vi "GLdrv_FILE_TRANS_SOUR.vi"(0 "Connection ID":T1, 5 "File Path":string, 11 "error in (no error)":errorcluster, 13 "Query(f)":bool) -> (4 "Connection ID Out":T1, 6 "File Path out":string, 15 "error out":errorcluster)   [LabVIEW 2017, in "GL860_Driver.lvlib"]
doc: "記録計本体内のファイルを転送します\nファイルの設定を行います\n例）　:FILE:TRNAS:SOUR \"MEM\\FOLDER\\ABCD.GBD”"
uses:
  GL860_Driver.lvlib
  ConnectionID.ctl
  GLdrv_RW.ctl
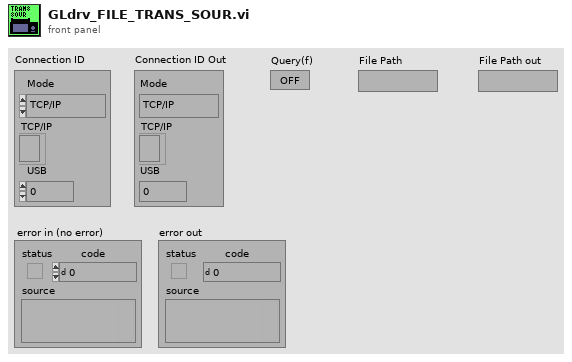
[diagram p1: front panel]
types:
  T1 = typedef "ConnectionID.ctl" = cluster{"Mode":enum16{"TCP/IP", "USB"}, "TCP/IP":refnum<k5>, "USB":i32}
  T2 = typedef "GLdrv_RW.ctl" = enum16{"Auto", "Read", "Write", "Buffer"}
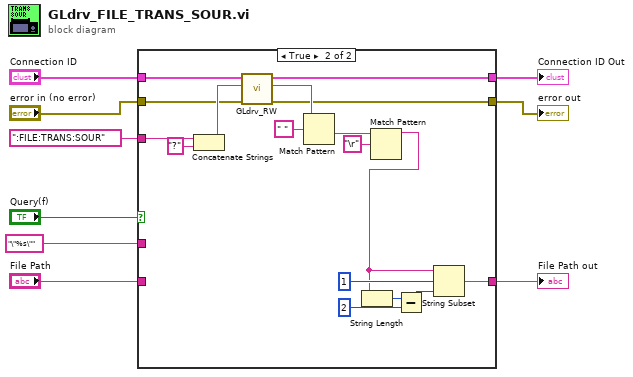
[diagram p0: block diagram]
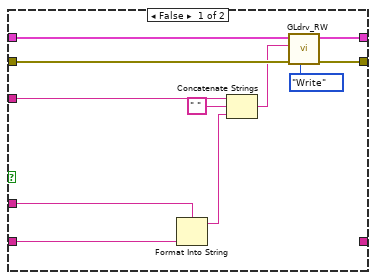
[diagram p2: hidden frame]
diagram:
  n1 = case shown="TRUE" "Query(f)" {
    tunnel: ":FILE:TRANS:SOUR" ("Command") -> [w20 w34]
    tunnel: [w15 w27] -> w9
    tunnel: [w17 w31] -> w8
    tunnel: "Connection ID" -> [w18 w32]
    tunnel: "error in (no error)" -> [w16 w28]
    tunnel: "File Path" -> [w11 _]
    tunnel: [_ w22] -> w1
    tunnel: "\"%s\"" ("Param") -> [w10 _]
    frame False {
      n2 = Format Into String(format string=w10, w11) -> (resulting string=w12:string)  [unwired: 2 in, 1 out]
      n3 = Concatenate Strings(w20, " " ("string"), w12) -> (w14:string)
      n4 = call "GLdrv_RW.vi"("Mode(read)"=GLdrv_RW."Write", "error in (no error)"=w16, "data in"=w14, "Connection ID"=w18) -> ("error out"=w15:errorcluster, "Connection ID Out"=w17:T1)  [unwired: 3 in, 3 out]
    }
    frame True {
      n5 = Concatenate Strings(w34, "?" ("string")) -> (w30:string)
      n6 = call "GLdrv_RW.vi"("error in (no error)"=w28, "data in"=w30, "Connection ID"=w32) -> ("error out"=w27:errorcluster, "data out"=w29:string, "Connection ID Out"=w31:T1)  [unwired: 4 in, 2 out]
      n7 = Match Pattern(string=w29, regular expression=" " ("search string/char (-)")) -> (after substring=w35:string)  [unwired: 4 out]
      n8 = Match Pattern(string=w35, regular expression="\r") -> (before substring=w21:string)  [unwired: 4 out]
      n9 = String Length(string=w21) -> (length=w24:i32)
      n10 = Subtract(x=w24, y=2) -> (x-y=w25:i32)
      n11 = String Subset(string=w21, offset (0)=1, length (rest)=w25) -> (substring=w22:string)
    }
  }
  "Connection ID Out" <- w8
  "error out" <- w9
  "File Path out" <- w1
